vi "DisableCell.vi"(0 "SingleValCol in":refnum<class "SingleValCol.lvclass">, 5 "Cell Position":T1, 7 "Table Data in":string[][](array[string]), 9 "Table CtlRef In":refnum<vi>, 11 "error in (no error)":errorcluster) -> (4 "SingleValCol out":refnum<class "SingleValCol.lvclass">, 8 "Table Data out":string[][](array[string]), 10 "Table CtlRef Out":refnum<vi>, 15 "error out":errorcluster)   [LabVIEW 2013, in "SingleValCol.lvclass"]
uses:
  SingleValCol.lvclass
  <vilib>/Utility/miscctls.llb/LVRowAndColumnTypeDef.ctl
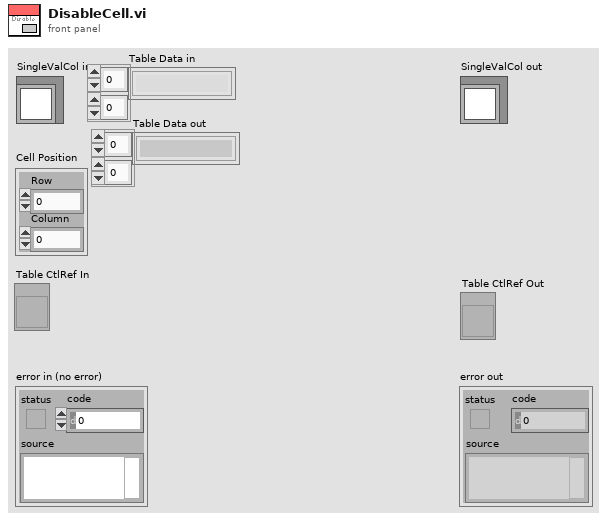
[diagram p1: front panel]
types:
  T1 = typedef "LVRowAndColumnTypeDef.ctl" = cluster{"Row":i32, "Column":i32}
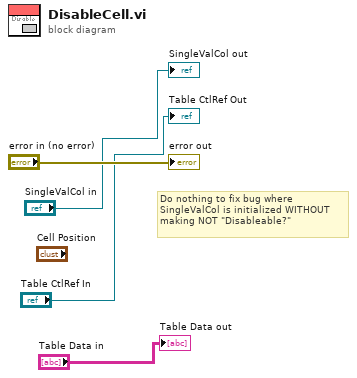
[diagram p0: block diagram]
diagram:
  # "Do nothing to fix bug where\nSingleValCol is initialized WITHOUT\nmaking NOT \"Disableable?\""
  "error out" <- "error in (no error)"
  "SingleValCol out" <- "SingleValCol in"
  "Table CtlRef Out" <- "Table CtlRef In"
  "Table Data out" <- "Table Data in"
